vi "init runtime data structures.vi"(8 "error in (no error)":errorcluster, 9 "data allocations":T1, 10 "alarms":T4[](array[typedef]), 11 "alarms module runtime in":refnum<class "alarms module runtime.lvclass">) -> (0 "error out":errorcluster, 3 "alarms module runtime out":refnum<class "alarms module runtime.lvclass">)   [LabVIEW 2013, in "alarms module runtime.lvclass"]
uses:
  alarms module runtime.lvclass
  configuration/alarm configuration.ctl
  <vilib>/NI/Tag Bus Module Framework/channel/TBM channel.lvclass
  configuration/alarm comparison.ctl
  configuration/compare type.ctl
  configuration/boolean operation.ctl
  <vilib>/NI/Tag Bus Module Framework/channel/data tables.ctl
  <vilib>/NI/Tag Bus/dictionary/data dictionary.lvclass
  <vilib>/NI/Tag Bus/dictionary table pair.ctl
  <vilib>/NI/Tag Bus/table/data table.ctl
  runtime alarm configuration.ctl
  runtime alarm comparison.ctl
  <vilib>/NI/Tag Bus/tag/Data Type.ctl
  <vilib>/NI/Tag Bus/tag/tag descriptor.lvclass/tag descriptor.ctl
  alarms module runtime.lvclass/alarms module runtime.ctl
  <vilib>/NI/Tag Bus/tag/read tag name.vi
  <vilib>/NI/Tag Bus/dictionary/locate tag.vi
  <vilib>/NI/Tag Bus/tag/tag descriptor.lvclass
  configuration/alarms module configuration.lvclass
  <vilib>/NI/Tag Bus/table/data table.lvlib
  <vilib>/NI/Tag Bus/tag bus.lvlib
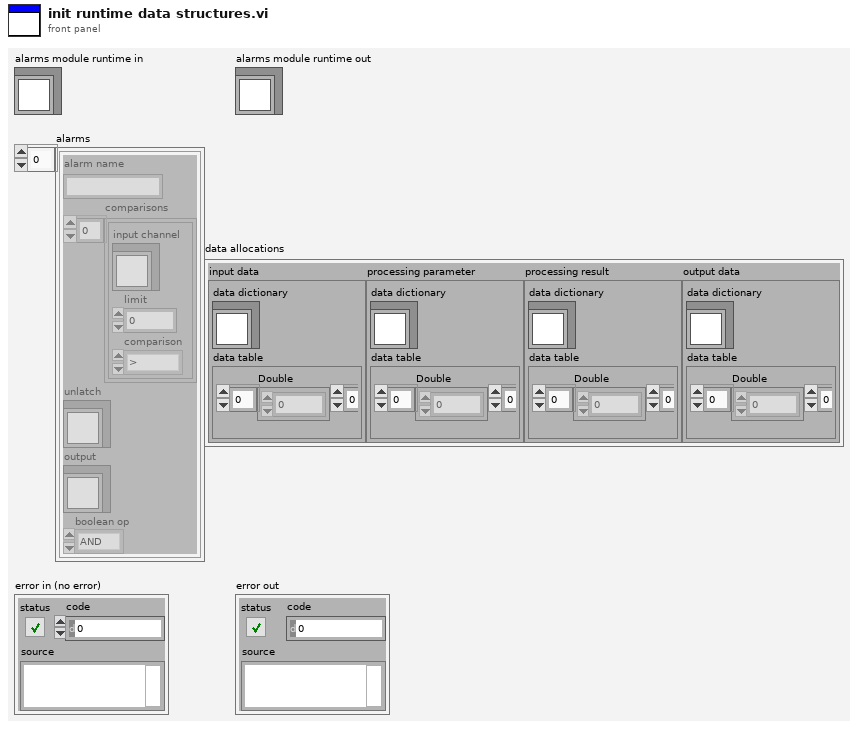
[diagram p1: front panel]
types:
  T1 = typedef "TBM channel.lvclass/data tables.ctl" = cluster{"input data":T2, "processing parameter":T2, "processing result":T2, "output data":T2}
  T2 = typedef "tag bus.lvlib/dictionary table pair.ctl" = cluster{"data dictionary":refnum<class "data dictionary.lvclass">, "data table":T3}
  T3 = typedef "tag bus.lvlib/data table.lvlib/data table.ctl" = cluster{"Double":dbl[], "Single":sgl[], "I64":i64[], "I32":i32[], "I16":i16[], "I8":i8[], "U64":u64[], "U32":u32[], "U16":u16[], "U8":u8[], "Boolean":bool[], "String":string[], "Array of Double":cluster{"DBL Array":dbl[]}[], "Array of Single":cluster{"SGL Array":sgl[]}[], "Array of I64":cluster{"I64 Array":i64[]}[], "Array of I32":cluster{"I32 Array":i32[]}[], "Array of I16":cluster{"I16 Array":i16[]}[], "Array of I8":cluster{"I8 Array":i8[]}[], "Array of U64":cluster{"U64 Array":u64[]}[], "Array of U32":cluster{"U32 Array":u32[]}[], "Array of U16":cluster{"U16 Array":u16[]}[], "Array of U8":cluster{"U8 Array":u8[]}[], "Array of Boolean":cluster{"Boolean Array":bool[]}[], "Array of String":cluster{"String Array":string[]}[]}
  T4 = typedef "alarms module configuration.lvclass/alarm configuration.ctl" = cluster{"alarm name":string, "comparisons":T5[], "unlatch":refnum<class "TBM channel.lvclass">, "output":refnum<class "TBM channel.lvclass">, "boolean op":T7}
  T5 = typedef "alarms module configuration.lvclass/alarm comparison.ctl" = cluster{"input channel":refnum<class "TBM channel.lvclass">, "limit":dbl, "comparison":T6}
  T6 = typedef "alarms module configuration.lvclass/compare type.ctl" = enum16{">", "<", ">=", "<=", "="}
  T7 = typedef "alarms module configuration.lvclass/boolean operation.ctl" = enum16{"AND", "OR"}
  T8 = typedef "alarms module runtime.lvclass/runtime alarm configuration.ctl" = cluster{"comparisons":T9[], "boolean op":T7, "unlatch index (bool)":i32, "output index (bool)":i32, "state":bool}
  T9 = typedef "alarms module runtime.lvclass/runtime alarm comparison.ctl" = cluster{"data type":T10, "index":i32, "limit":dbl, "comparison":T6}
  T10 = typedef "tag bus.lvlib/tag descriptor.lvclass/Data Type.ctl" = enum16{"Double", "Single", "I64", "I32", "I16", "I8", "U64", "U32", "U16", "U8", "Boolean", "String", "Array of Double", "Array of Single", "Array of I64", "Array of I32", "Array of I16", "Array of I8", "Array of U64", "Array of U32", "Array of U16", "Array of U8", "Array of Boolean", "Array of String"}
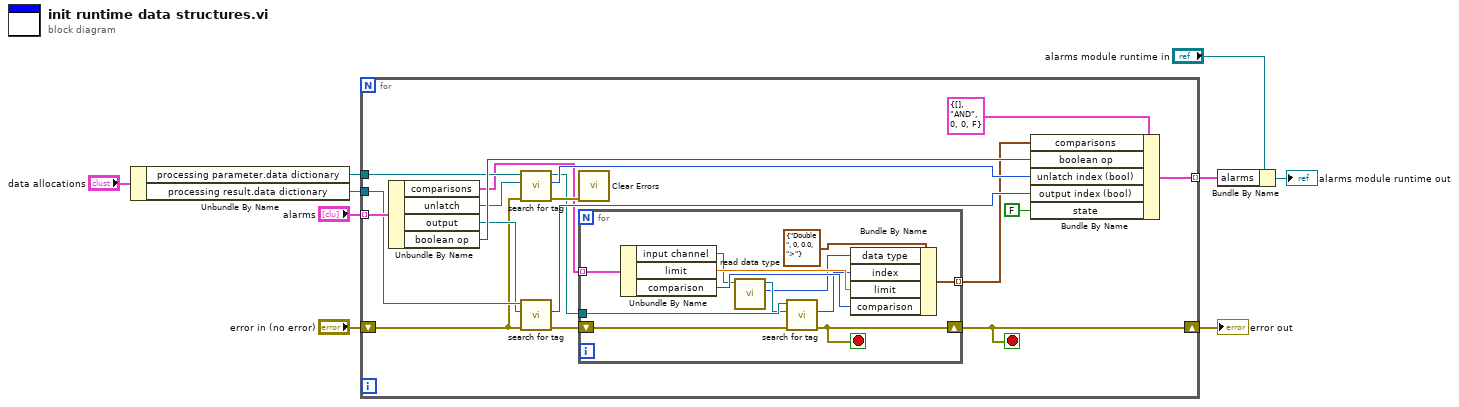
[diagram p0: block diagram]
diagram:
  n1 = Unbundle By Name("data allocations") -> ("processing parameter.data dictionary"=w1:refnum<class "data dictionary.lvclass">, "processing result.data dictionary"=w2:refnum<class "data dictionary.lvclass">)
  n2 = for {
    shift-right: [w23] -> w6
    shift-left: "error in (no error)" -> [w17]
    tunnel: "alarms" -> [w27] mode=indexing
    tunnel: [w24] -> w3 mode=indexing
    tunnel: w2 -> [w20]
    tunnel: w1 -> [w14]
    stop <- w23 stop-if-true
    n3 = Unbundle By Name(w27) -> ("comparisons"=w12:T5[], "unlatch"=w13:refnum<class "TBM channel.lvclass">, "output"=w19:refnum<class "TBM channel.lvclass">, "boolean op"=w22:T7)
    n4 = call <vilib>:"search for tag.vi"("error in"=w17, "system tag"=w13, "data dictionary in"=w14) -> ("error out"=w16:errorcluster, "index"=w15:i32, "data dictionary out"=w10:refnum<class "data dictionary.lvclass">)  [unwired: 6 in]
    n5 = call <vilib>:"search for tag.vi"("error in"=w17, "system tag"=w19, "data dictionary in"=w20) -> ("error out"=w21:errorcluster, "index"=w18:i32)  [unwired: 6 in, 1 out]
    n6 = call <vilib>:"Clear Errors.vi"("error in (no error)"=w16) -> ()  [unwired: 6 in, 1 out]
    n7 = for {
      shift-right: [w31] -> w23
      shift-left: w21 -> [w34]
      tunnel: w12 -> [w39] mode=indexing
      tunnel: [w37] -> w11 mode=indexing
      tunnel: w10 -> [w33]
      stop <- w31 stop-if-true
      n8 = Unbundle By Name(w39) -> ("input channel"=w30:refnum<class "TBM channel.lvclass">, "limit"=w35:dbl, "comparison"=w36:T6)
      n9 = call <vilib>:"read data type.vi"("system tag in"=w30) -> ("data type"=w28:T10, "system tag out"=w29:refnum<class "TBM channel.lvclass">)  [unwired: 8 in, 1 out]
      n10 = call <vilib>:"search for tag.vi"("error in"=w34, "system tag"=w29, "data dictionary in"=w33) -> ("error out"=w31:errorcluster, "index"=w32:i32)  [unwired: 6 in, 1 out]
      n11 = Bundle By Name(cluster=T9 {"data type"=enum."Double", "index"=0, "limit"=0.0, "comparison"=enum.">"} ("alarm cfg"), "data type"=w28, "index"=w32, "limit"=w35, "comparison"=w36) -> (w37:T9)
    }
    n12 = Bundle By Name(cluster=T8 {"comparisons"=[], "boolean op"=enum."AND", "unlatch index (bool)"=0, "output index (bool)"=0, "state"=FALSE} ("alarm config"), "comparisons"=w11, "boolean op"=w22, "unlatch index (bool)"=w15, "output index (bool)"=w18, "state"=FALSE) -> (w24:T8)
  }
  "error out" <- w6
  n13 = Bundle By Name(cluster="alarms module runtime in", "alarms"=w3) -> (→"alarms module runtime out":refnum<class "alarms module runtime.lvclass">)
